vi "set_ref_clus.vi"(6 "cluster_ref":T1, 8 "he_level":dbl, 9 "bypass_valve_opening":dbl, 10 "run_valve_opening":dbl, 11 "status":bool) -> ()   [LabVIEW 2019]
uses:
  cluster_ref_fridge_valve.ctl
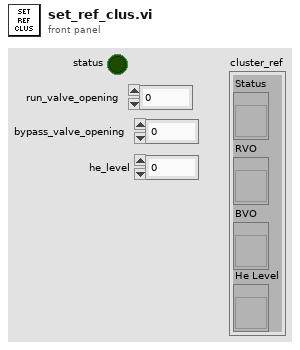
[diagram p1: front panel]
types:
  T1 = typedef "cluster_ref_fridge_valve.ctl" = cluster{"Status":refnum<vi>, "RVO":refnum<vi>, "BVO":refnum<vi>, "He Level":refnum<vi>}
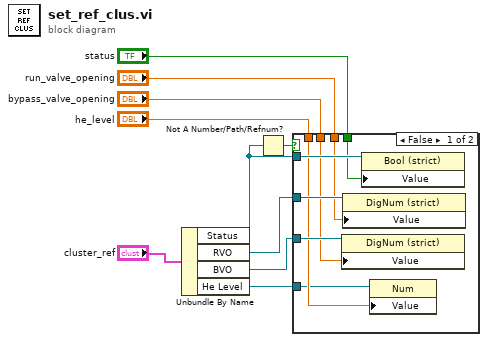
[diagram p0: block diagram]
diagram:
  n1 = Unbundle By Name("cluster_ref") -> ("Status"=w7:refnum<vi>, "RVO"=w8:refnum<vi>, "BVO"=w9:refnum<vi>, "He Level"=w1:refnum<vi>)
  n2 = Not A Number/Path/Refnum?(number/path/refnum=w7) -> (NaN/Path/Refnum?=w10:bool)
  n3 = case shown="False" w10 {
    tunnel: w8 -> [w18 _]
    tunnel: w9 -> [w17 _]
    tunnel: w7 -> [w16 _]
    tunnel: "status" -> [w15 _]
    tunnel: "run_valve_opening" -> [w14 _]
    tunnel: "bypass_valve_opening" -> [w13 _]
    tunnel: "he_level" -> [w12 _]
    tunnel: w1 -> [w11 _]
    frame False {
      n4 = property class="DigNum (strict)"(reference=w17, "Value"=w13) -> ()  [unwired: 1 in, 2 out]
      n5 = property class="DigNum (strict)"(reference=w18, "Value"=w14) -> ()  [unwired: 1 in, 2 out]
      n6 = property class="Bool (strict)"(reference=w16, "Value"=w15) -> ()  [unwired: 1 in, 2 out]
      n7 = property class="Num"(reference=w11, "Value"=w12) -> ()  [unwired: 1 in, 2 out]
    }
    frame True {
    }
  }
